vi "Dsc_Board_Man_Dlg.vi"(8 "error in":errorcluster) -> (0 "error out":errorcluster)   [LabVIEW 2014, in "Dsc_Board_Dlg.lvlib"]
uses:
  Dsc_Board_Dlg.lvlib
  <vilib>/Utility/miscctls.llb/LVRowAndColumnTypeDef.ctl
  DataBase/DataBase.lvlib
  DetectElecrodes/DetectElectros.lvlib
panel:
  in  "退出":bool
  in  "删除":bool
  in  "修改":bool
  in  "新增":bool
  in  "采集卡管理":i32(listbox)
  in  "OK":bool
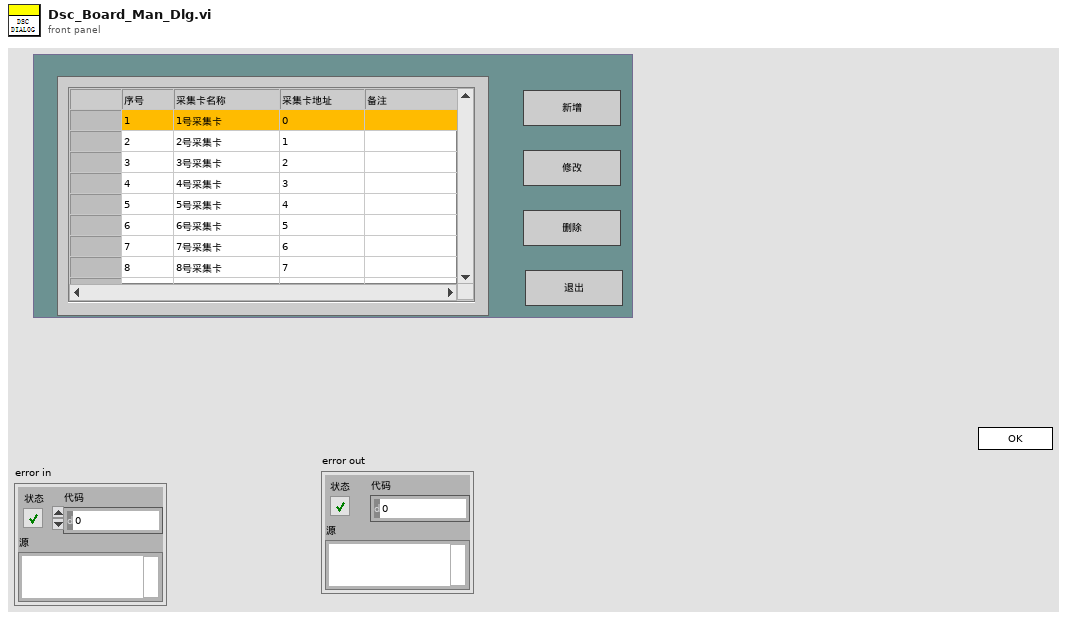
[diagram p1: front panel]
types:
  T1 = enum32{"invalid app kind", "Development System", "Run Time System", "Student Edition", "Embedded LabVIEW", "Evaluation", "Custom"}
  T2 = enum32{"Invalid", "Standard", "Closed", "Hidden", "Minimized", "Maximized"}
  T3 = typedef "LVPoint32TypeDef.ctl" = cluster{"Horizontal":i32, "Vertical":i32}
  T4 = typedef "LVRowAndColumnTypeDef.ctl" = cluster{"Row":i32, "Column":i32}
  T5 = cluster{"Core":cluster{"Current VI Reference":refnum<vi>, "Close Panel on Exit?":bool}, "Your Boolean data":bool, "Your string data":string, "行列":T4}
  T6 = cluster{"Current VI Reference":refnum<vi>, "Close Panel on Exit?":bool}
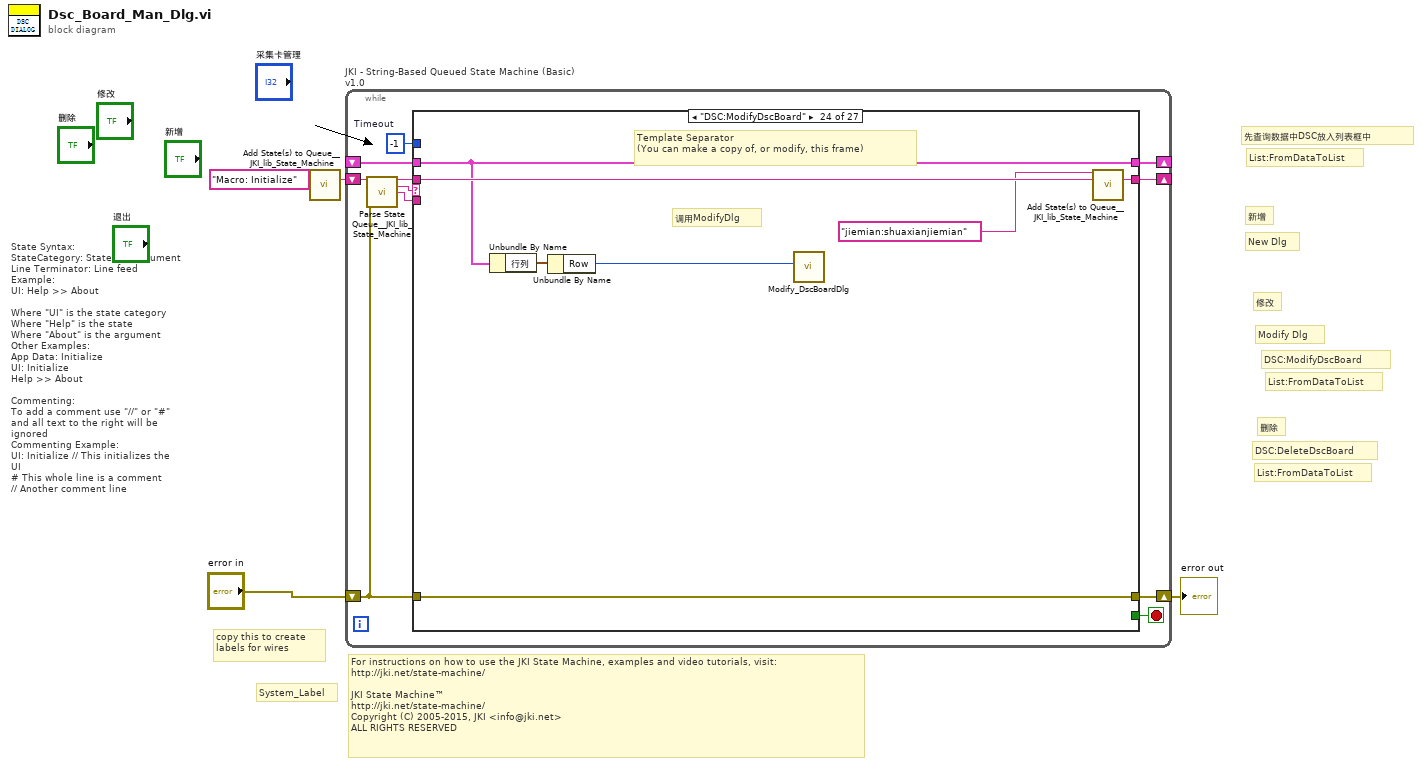
[diagram p0: block diagram]
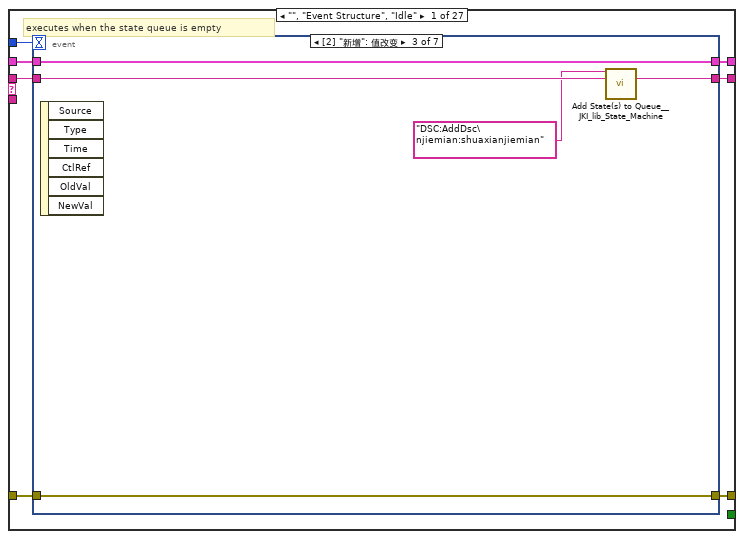
[diagram p2: hidden frame]
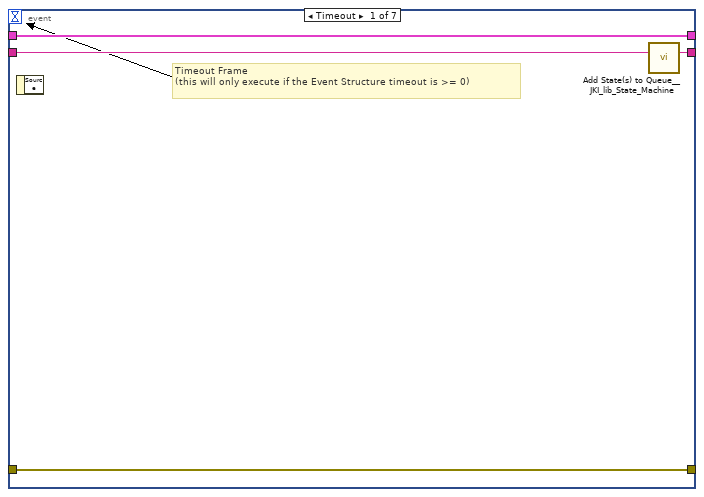
[diagram p3: hidden frame]
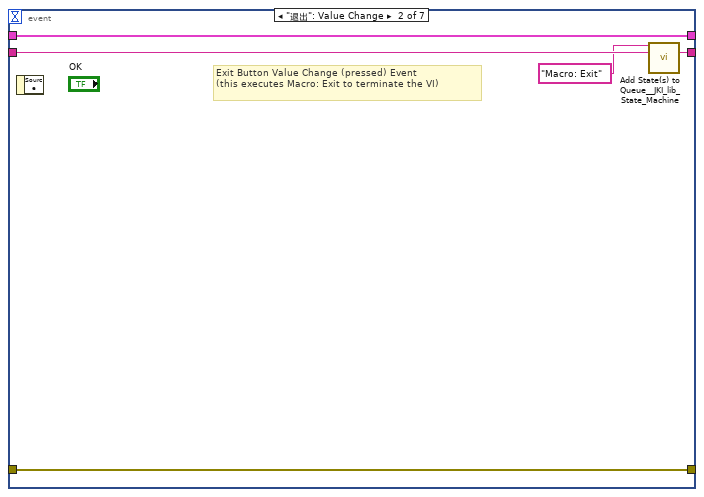
[diagram p4: hidden frame]
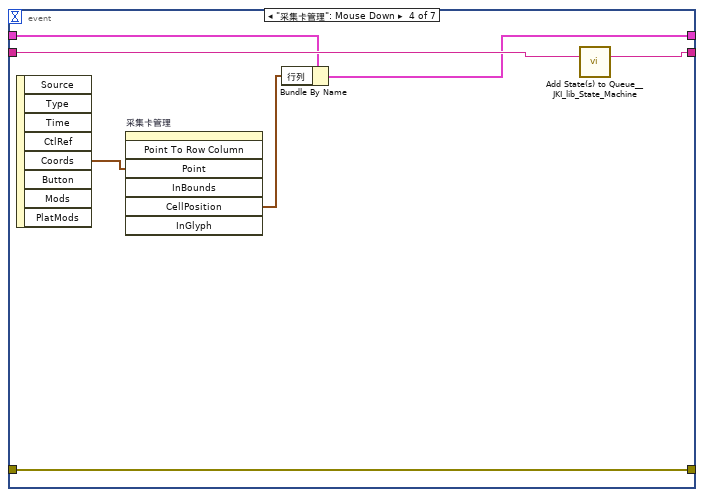
[diagram p5: hidden frame]
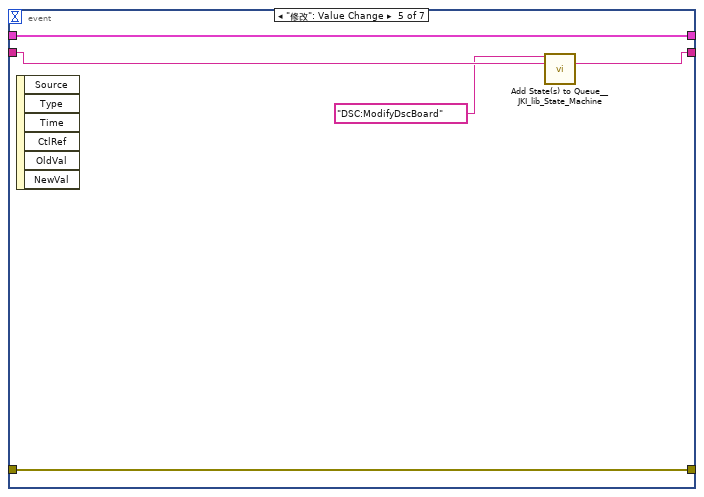
[diagram p6: hidden frame]
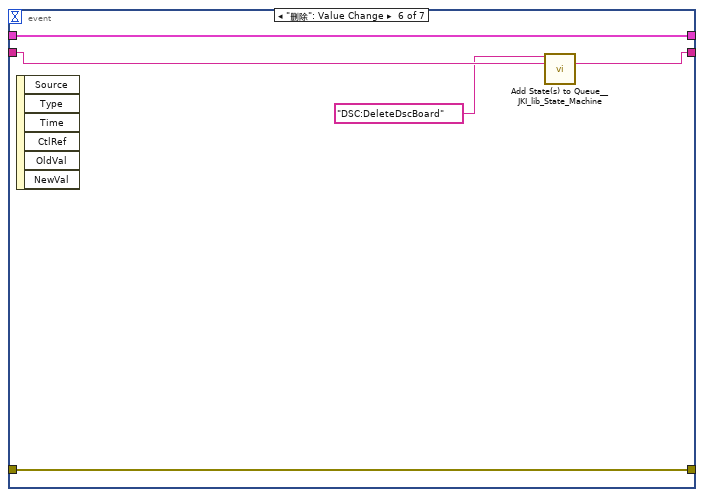
[diagram p7: hidden frame]
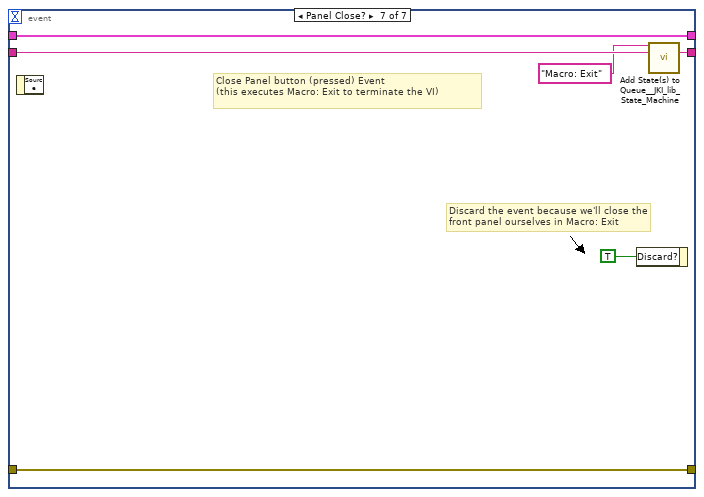
[diagram p8: hidden frame]
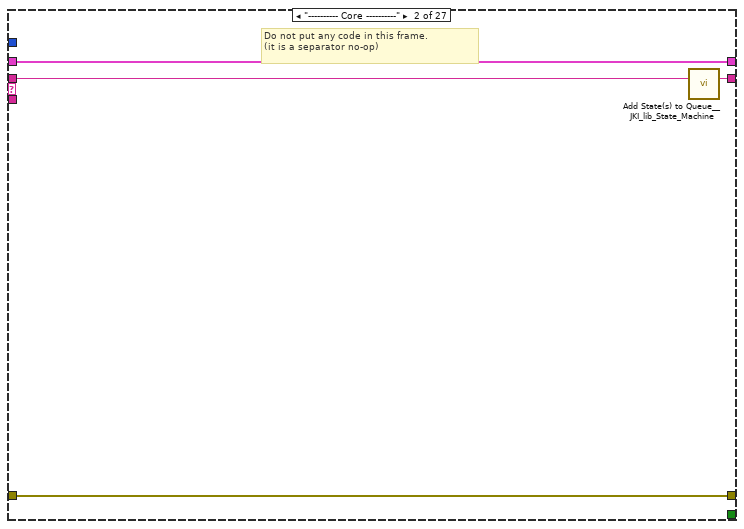
[diagram p9: hidden frame]
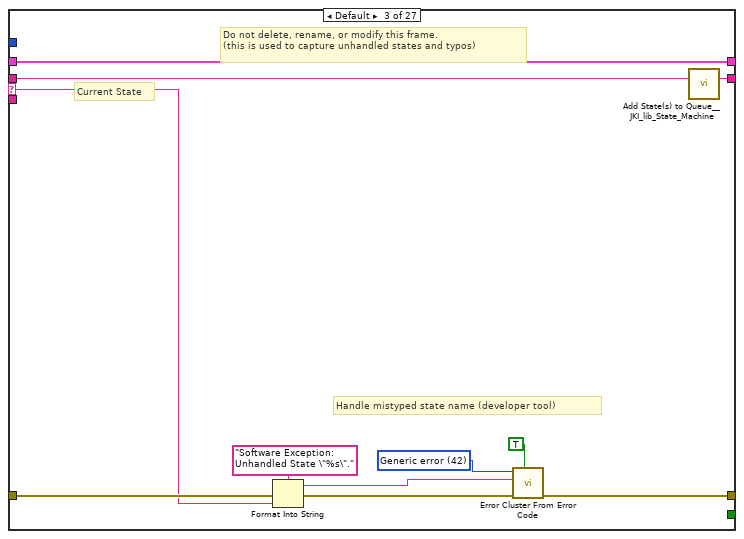
[diagram p10: hidden frame]
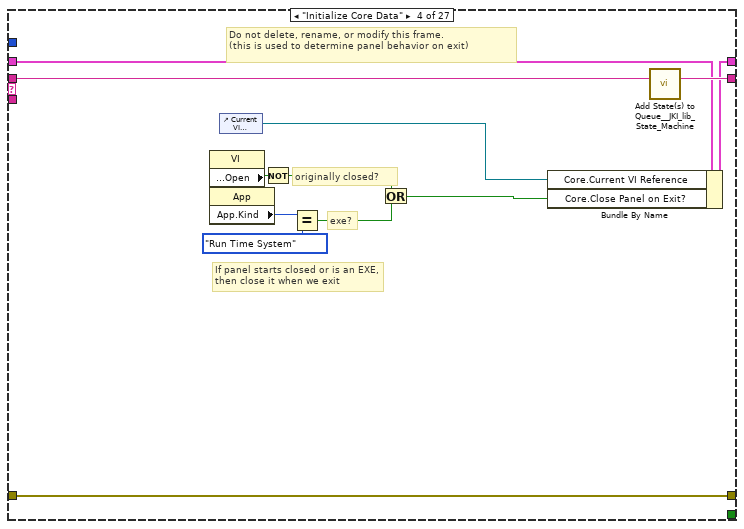
[diagram p11: hidden frame]
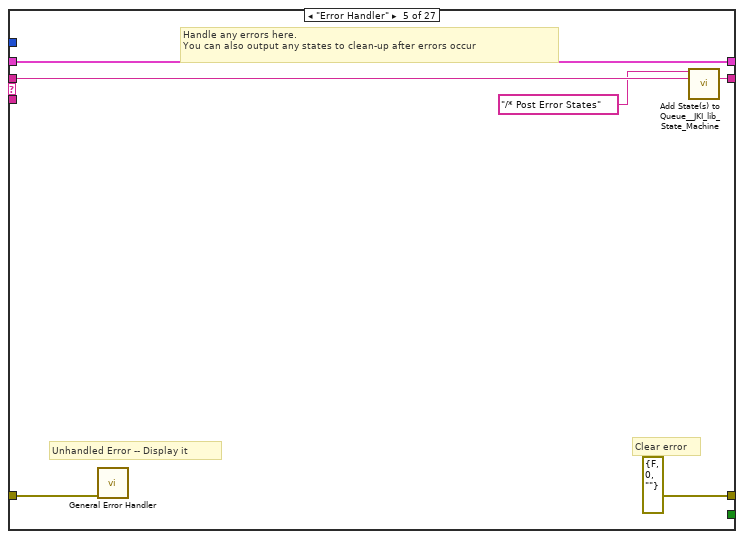
[diagram p12: hidden frame]
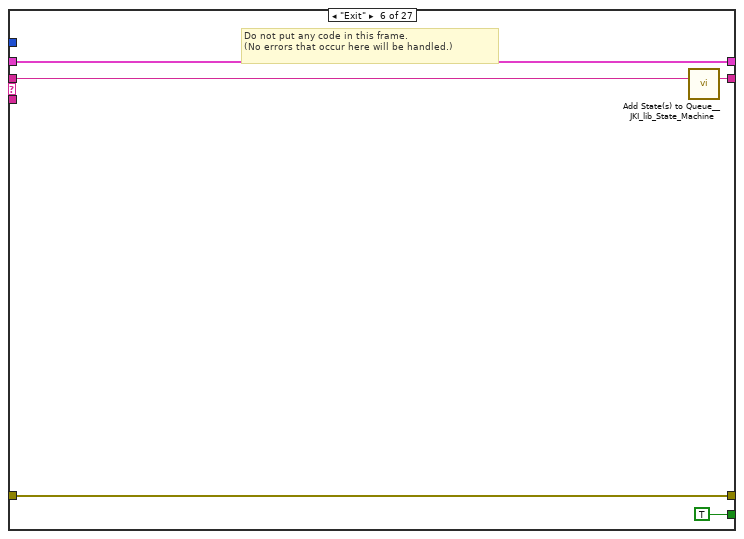
[diagram p13: hidden frame]
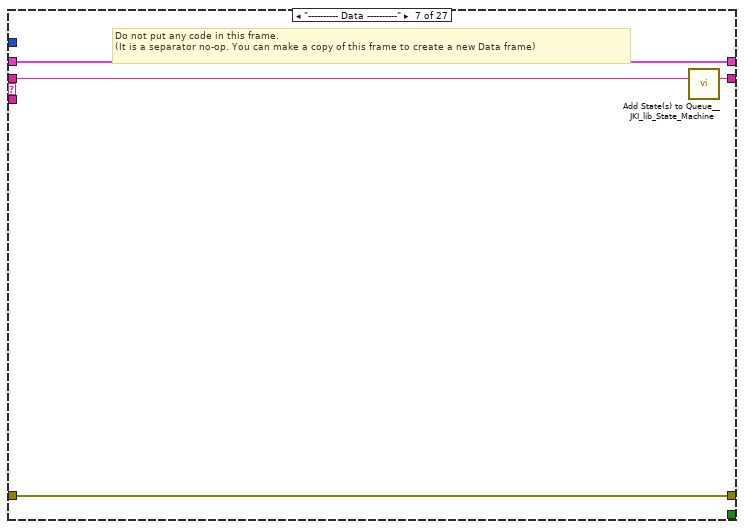
[diagram p14: hidden frame]
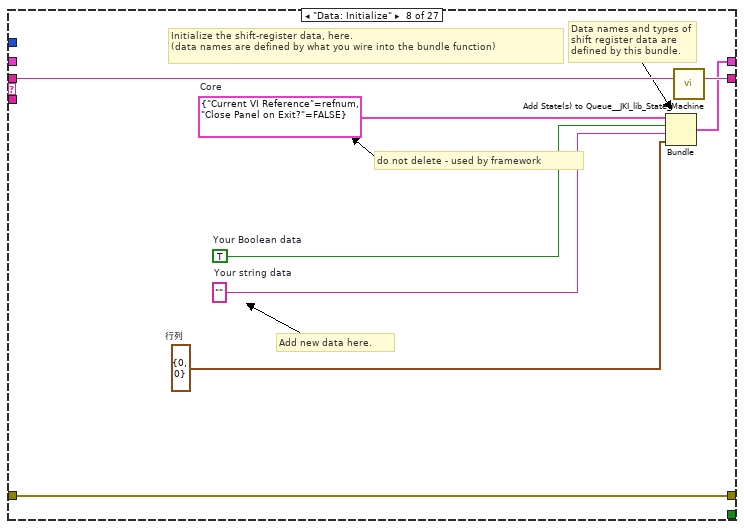
[diagram p15: hidden frame]
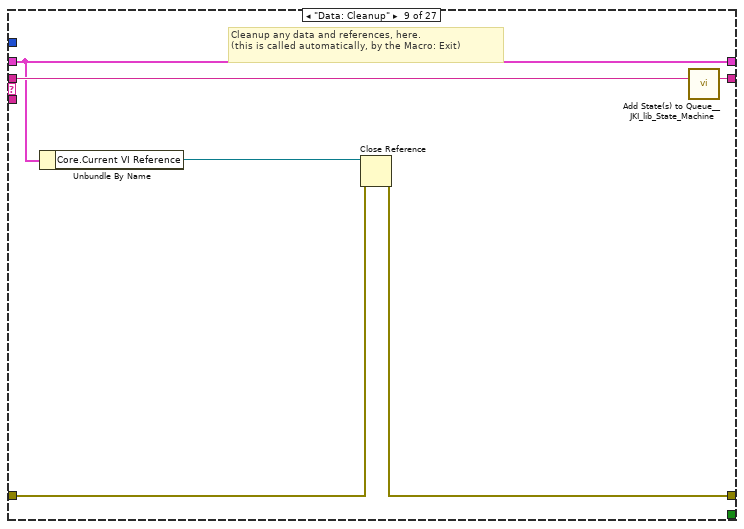
[diagram p16: hidden frame]
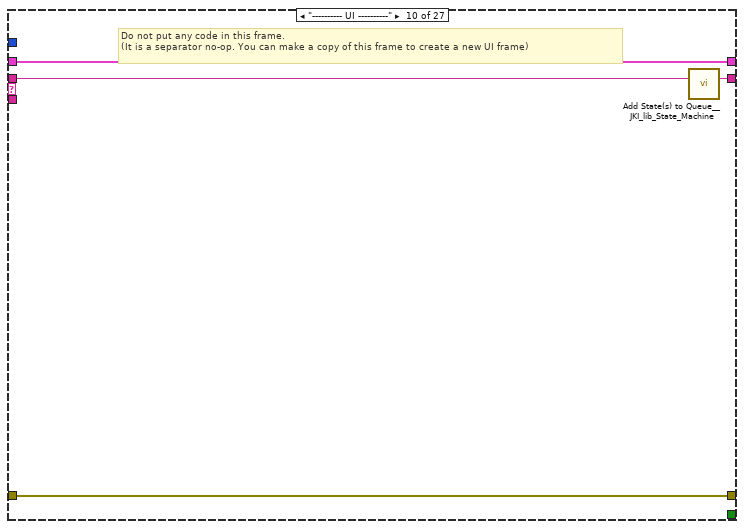
[diagram p17: hidden frame]
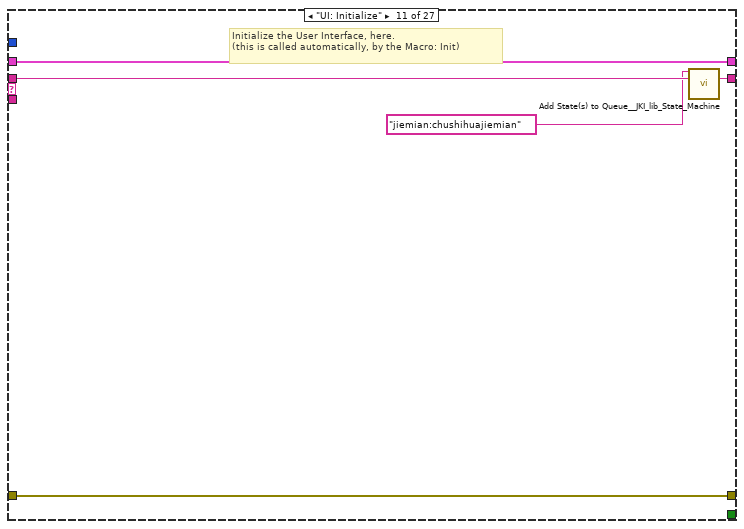
[diagram p18: hidden frame]
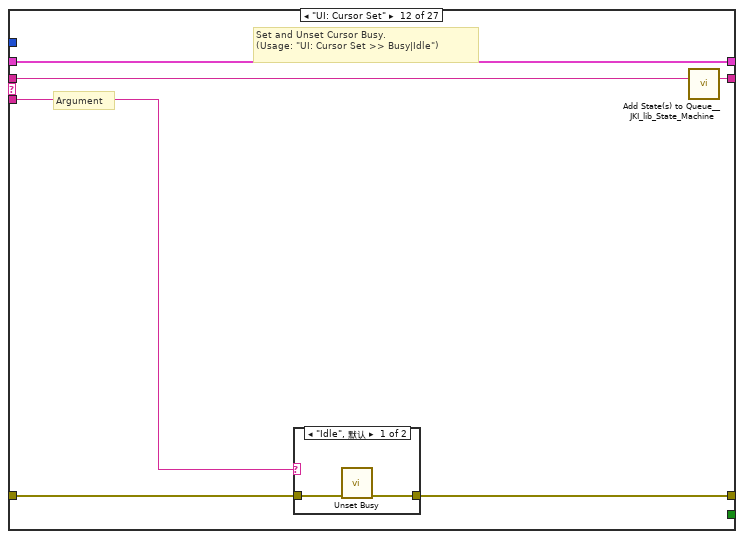
[diagram p19: hidden frame]
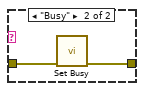
[diagram p20: hidden frame]
diagram:
  # "List:FromDataToList"
  # "DSC:DeleteDscBoard"
  # "删除"
  # "List:FromDataToList"
  # "DSC:ModifyDscBoard"
  # "Modify Dlg"
  # "修改"
  # "New Dlg"
  # "List:FromDataToList"
  # "先查询数据中DSC放入列表框中"
  # "新增"
  # "For instructions on how to use the JKI State Machine, examples and video tutorials, visit:\nhttp://jki.net/state-machine/\n\nJKI State Machine™\nhttp://jki.net/state-machine/\nCopyright (C) 2005-2015, JKI <info@jki.net>\nALL RIGHTS RESERVED"
  # "State Syntax:\nStateCategory: State >> Argument\nLine Terminator: Line feed\nExample:\nUI: Help >> About\n\nWhere \"UI\" is the state category\nWhere \"Help\" is the state\nWhere \"About\" is the argument\nOther Examples:\nApp Data: Initialize\nUI: Initialize\nHelp >> About\n\nCommenting:\nTo add a comment use \"//\" or \"#\" and all text to the right will be ignored\nCommenting Example:\nUI: Initialize // This initializes the UI\n# This whole line is a comment\n// Another comment line"
  # "copy this to create labels for wires"
  # "System_Label"
  n1 = call <vilib>:"Add State(s) to Queue__JKI_lib_State_Machine.vi"("State(s) in (\"\")"="Macro: Initialize") -> ("States Out"=w4:string)  [unwired: 14 in]
  n2 = while "JKI - String-Based Queued State Machine (Basic) v1.0" {
    shift-right: [w8] -> _
    shift-left: _ -> [w7]
    shift-right: [w11] -> w2
    shift-left: "error in" -> [w5]
    shift-right: [w10] -> _
    shift-left: w4 -> [w12]
    stop <- w9 stop-if-true
    w6 = -1  # Timeout
    n3 = call <vilib>:"Parse State Queue__JKI_lib_State_Machine.vi"("State Queue"=w12, "Error In (no error)"=w5) -> ("Remaining States"=w14:string, "Current State"=w15:string, "Arguments"=w13:string)  [unwired: 11 in]
    n4 = case shown="\"DSC:ModifyDscBoard\"" w15 {
      selector: w15 -> [_ _ w64 _ _ _ _ _ _ _ _ _ _ _ _ _ _ _ _ _ _ _ _ _ _ _ _]
      tunnel: w14 -> [w22 w63 w68 w86 w92 w97 w101 w109 w115 w119 w124 w130 w141 w167 w172 w182 w186 w197 w206 w215 w219 w223 w233 w240 w244 w248 w252]
      tunnel: w13 -> [_ _ _ _ _ _ _ _ _ _ _ w125 w135 _ _ _ _ _ _ _ _ _ _ _ _ _ _]
      tunnel: w7 -> [w20 w60 w66 w77 w89 w95 w98 _ w110 w116 w122 w128 w137 w164 w169 w179 w183 w194 w203 w212 w216 w220 w231 w237 w241 w245 w249]
      tunnel: [w19 w61 w70 w83 errorcluster {"status"=FALSE, "code"=0, "source"=""} ("error out") w94 w99 w106 w111 w117 w121 w126 w138 w165 w170 w180 w184 w195 w204 w213 w217 w221 w225 w238 w242 w246 w250] -> w11
      tunnel: w5 -> [w18 w61 w69 w83 w88 w94 w99 w106 w112 w117 w121 w127 w139 w165 w170 w180 w184 w195 w204 w213 w217 w221 w226 w238 w242 w246 w250]
      tunnel: [w21 w62 w67 w85 w91 w96 w100 w108 w114 w118 w123 w129 w140 w166 w171 w181 w185 w196 w205 w214 w218 w222 w232 w239 w243 w247 w251] -> w10
      tunnel: [_ _ _ _ _ TRUE _ _ _ _ _ _ _ _ _ _ _ _ _ _ _ _ _ _ _ _ _] -> w9
      tunnel: [w17 w60 w66 w84 w89 w95 w98 w107 w110 w116 w122 w128 w137 w164 w169 w179 w183 w194 w203 w212 w216 w220 w231 w237 w241 w245 w249] -> w8
      tunnel: w6 -> [w16 _ _ _ _ _ _ _ _ _ _ _ _ _ _ _ _ _ _ _ _ _ _ _ _ _ _]
      frame "", "Event Structure", "Idle" {
        # "executes when the state queue is empty"
        n5 = event shown="[2] \"新增\": 值改变" {
          selector: _ -> [_ _ _ _ _ _ _]
          dyn-events: _ -> [_ _ _ _ _ _ _]
          timeout: w16 -> [_ _ _ _ _ _ _]
          tunnel: w22 -> [w26 w31 w35 w42 w46 w51 w59]
          tunnel: [w25 w30 w36 w43 w48 w53 w58] -> w21
          tunnel: w20 -> [w23 w28 w33 w38 w47 w52 w56]
          tunnel: [w24 w29 w34 w40 w44 w49 w57] -> w19
          tunnel: w18 -> [w24 w29 w34 w40 w44 w49 w57]
          tunnel: [w23 w28 w33 w37 w47 w52 w56] -> w17
          event Timeout {
            # "Timeout Frame\n(this will only execute if the Event Structure timeout is >= 0)"
            n6 = event-data() -> ()  [unwired: 1 in, 1 out]
            n7 = call <vilib>:"Add State(s) to Queue__JKI_lib_State_Machine.vi"("State(s) in (\"\")"=w26) -> ("States Out"=w25:string)  [unwired: 14 in]
          }
          event "退出": Value Change {
            # "Exit Button Value Change (pressed) Event\n(this executes Macro: Exit to terminate the VI)"
            n8 = event-data() -> ()  [unwired: 1 in, 1 out]
            n9 = call <vilib>:"Add State(s) to Queue__JKI_lib_State_Machine.vi"("State(s) in Front (\"\")"="Macro: Exit", "State(s) in (\"\")"=w31) -> ("States Out"=w30:string)  [unwired: 13 in]
          }
          event "新增": Value Change {
            n10 = event-data() -> ()  [unwired: 1 in, 6 out]
            n11 = call <vilib>:"Add State(s) to Queue__JKI_lib_State_Machine.vi"("State(s) in Front (\"\")"="DSC:AddDsc\njiemian:shuaxianjiemian", "State(s) in (\"\")"=w35) -> ("States Out"=w36:string)  [unwired: 13 in]
          }
          event "采集卡管理": Mouse Down {
            n12 = event-data() -> ("Coords"=w41:T3)  [unwired: 1 in, 7 out]
            n13 = invoke on="采集卡管理" class="MCListbox (严格)" method="Point To Row Column"("Point"=w41) -> ("CellPosition"=w39:T4)  [unwired: 6 in, 6 out]
            n14 = Bundle By Name(cluster=w38, "行列"=w39) -> (w37:T5)
            n15 = call <vilib>:"Add State(s) to Queue__JKI_lib_State_Machine.vi"("State(s) in (\"\")"=w42) -> ("States Out"=w43:string)  [unwired: 14 in]
          }
          event "修改": Value Change {
            n16 = event-data() -> ()  [unwired: 1 in, 6 out]
            n17 = call <vilib>:"Add State(s) to Queue__JKI_lib_State_Machine.vi"("State(s) in Front (\"\")"="DSC:ModifyDscBoard", "State(s) in (\"\")"=w46) -> ("States Out"=w48:string)  [unwired: 13 in]
          }
          event "删除": Value Change {
            n18 = event-data() -> ()  [unwired: 1 in, 6 out]
            n19 = call <vilib>:"Add State(s) to Queue__JKI_lib_State_Machine.vi"("State(s) in Front (\"\")"="DSC:DeleteDscBoard", "State(s) in (\"\")"=w51) -> ("States Out"=w53:string)  [unwired: 13 in]
          }
          event Panel Close? {
            # "Discard the event because we'll close the front panel ourselves in Macro: Exit"
            # "Close Panel button (pressed) Event\n(this executes Macro: Exit to terminate the VI)"
            n20 = event-data() -> ()  [unwired: 1 in, 1 out]
            n21 = event-data("Discard?"=TRUE) -> ()  [unwired: 1 in, 1 out]
            n22 = call <vilib>:"Add State(s) to Queue__JKI_lib_State_Machine.vi"("State(s) in Front (\"\")"="Macro: Exit", "State(s) in (\"\")"=w59) -> ("States Out"=w58:string)  [unwired: 13 in]
          }
        }
      }
      frame "---------- Core ----------" {
        # "Do not put any code in this frame.\n(it is a separator no-op)"
        n23 = call <vilib>:"Add State(s) to Queue__JKI_lib_State_Machine.vi"("State(s) in (\"\")"=w63) -> ("States Out"=w62:string)  [unwired: 14 in]
      }
      frame Default {
        w73 = 42 items=["No error", "Argument error", "Memory is full", "Out of zone", "End of file", "File already open", "Generic file I/O error", "File not found", "File permission error", "Disk is full", "Duplicate path", "Too many files open", "System feature not enabled", "Resource file not found", "Cannot add resource", "Resource not found", "Image not found", "Image memory error", "Pen does not exist", "Config type invalid", "Config token not found", "Config parse error", "Config memory error", "Bad external code format", "Bad external code offset", "External code not present", "Null window", "Destroy window error", "Null menu", "Print aborted", "Bad print record", "Print driver error", "Windows error during printing", "Memory error during printing", "Print dialog error", "Generic print error", "Invalid device refnum", "Device not found", "Device parameter error", "Device unit error", "Cannot open device", "Device call aborted", "Generic error", "Cancelled by user", "Object ID too low", "Object ID too high", "Object not in heap", "Unknown heap", "Unknown object (invalid DefProc)", "Unknown object (DefProc not in table)", "Message out of range", "Invalid (null) method", "Unknown message", "Manager call not supported", "Bad address", "Network operation in progress", "Network operation timed out", "Connection is busy", "Network attribute not supported", "Network error", "Address in use", "System out of memory", "Connection aborted", "Connection refused", "Not connected", "Already connected", "Connection closed", "Initialization error (interapplication manager)", "Bad occurrence", "Wait on unbound occurrence handler", "Occurrence queue overflow", "Datalog type conflict", "Unused", "Unrecognized type (interapplication manager)", "Memory corrupt", "Failed to make temporary DLL", "Old CIN version", "Drag socket not found", "Failed to load drop-object", "Failed to register OLE object", "Failed to release OLE object", "Format specifier type mismatch", "Unknown format specifier", "Too few format specifiers", "Too many format specifiers", "Scan failed", "Newer CIN version", "Error converting to variant", "Runtime menu error", "Password tampered", "Variant attribute not found", "Incompatible variant data type", "Event data is not available", "Event Store is not present", "Occurrence is not found", "Event Queue is not created", "Event info is not available", "Refnum passed is NULL", "Error retrieving Class GUID", "Error retrieving CoClass GUID", "Error retrieving TypeLib GUID.", "Bad built application magic bytes.", "Specific driver is different from the specific driver associated with the Logical Name.", "There is no session opened to the class driver.", "Max Error", "MAX - Error with config objects", "MAX - Error loading configuration", "MAX - Group not supported"]
        # "Current State"
        # "Do not delete, rename, or modify this frame.\n(this is used to capture unhandled states and typos)"
        # "Handle mistyped state name (developer tool)"
        n24 = Format Into String(format string="Software Exception: Unhandled State \"%s\"." ("message"), error in=w69, w64) -> (resulting string=w72:string, error out=w71:errorcluster)  [unwired: 1 in]
        n25 = call <vilib>:"Error Cluster From Error Code.vi"("show call chain? (False)"=TRUE, "error in (no error)"=w71, "error message (\"\")"=w72, "error code (0)"=w73) -> ("error out"=w70:errorcluster)  [unwired: 5 in]
        n26 = call <vilib>:"Add State(s) to Queue__JKI_lib_State_Machine.vi"("State(s) in (\"\")"=w68) -> ("States Out"=w67:string)  [unwired: 14 in]
      }
      frame "Initialize Core Data" {
        # "Do not delete, rename, or modify this frame.\n(this is used to determine panel behavior on exit)"
        # "originally closed?"
        # "exe?"
        # "If panel starts closed or is an EXE, then close it when we exit"
        n27 = property class="VI"() -> ("Front Panel.Open"=w82:bool)  [unwired: 2 in, 2 out]
        n28 = property class="App"() -> ("App.Kind"=w81:T1)  [unwired: 2 in, 2 out]
        n29 = control-ref of="Current VI Reference"() -> (w75:refnum<vi>)
        n30 = Not(x=w82) -> (.not. x?=w79:bool)
        n31 = Equal?(x=w81, y=T1."Run Time System" ("Application:Kind")) -> (x = y?=w78:bool)
        n32 = Or(x=w79, y=w78) -> (x .or. y?=w76:bool)
        n33 = Bundle By Name(cluster=w77, "Core.Current VI Reference"=w75, "Core.Close Panel on Exit?"=w76) -> (w84:T5)
        n34 = call <vilib>:"Add State(s) to Queue__JKI_lib_State_Machine.vi"("State(s) in (\"\")"=w86) -> ("States Out"=w85:string)  [unwired: 14 in]
      }
      frame "Error Handler" {
        # "Unhandled Error -- Display it"
        # "Handle any errors here.\nYou can also output any states to clean-up after errors occur"
        # "Clear error"
        n35 = call <vilib>:"General Error Handler.vi"("error in (no error)"=w88) -> ()  [unwired: 10 in, 5 out]
        n36 = call <vilib>:"Add State(s) to Queue__JKI_lib_State_Machine.vi"("State(s) in Front (\"\")"="/* Post Error States", "State(s) in (\"\")"=w92) -> ("States Out"=w91:string)  [unwired: 13 in]
      }
      frame "Exit" {
        # "Do not put any code in this frame.\n(No errors that occur here will be handled.)"
        n37 = call <vilib>:"Add State(s) to Queue__JKI_lib_State_Machine.vi"("State(s) in (\"\")"=w97) -> ("States Out"=w96:string)  [unwired: 14 in]
      }
      frame "---------- Data ----------" {
        # "Do not put any code in this frame.\n(It is a separator no-op. You can make a copy of this frame to create a new Data frame)"
        n38 = call <vilib>:"Add State(s) to Queue__JKI_lib_State_Machine.vi"("State(s) in (\"\")"=w101) -> ("States Out"=w100:string)  [unwired: 14 in]
      }
      frame "Data: Initialize" {
        w102 = T4 {"Row"=0, "Column"=0}  # 行列
        w103 = T6 {"Current VI Reference"=refnum, "Close Panel on Exit?"=FALSE}  # Core
        w105 = TRUE  # Your Boolean data
        w104 = ""  # Your string data
        # "do not delete - used by framework"
        # "Add new data here."
        # "Data names and types of shift register data are defined by this bundle."
        # "Initialize the shift-register data, here.\n(data names are defined by what you wire into the bundle function)"
        n39 = Bundle("Core"=w103, "Your Boolean data"=w105, "Your string data"=w104, "行列"=w102) -> (w107:T5)  [unwired: 1 in]
        n40 = call <vilib>:"Add State(s) to Queue__JKI_lib_State_Machine.vi"("State(s) in (\"\")"=w109) -> ("States Out"=w108:string)  [unwired: 14 in]
      }
      frame "Data: Cleanup" {
        # "Cleanup any data and references, here.\n(this is called automatically, by the Macro: Exit)"
        n41 = Unbundle By Name(w110) -> ("Core.Current VI Reference"=w113:refnum<vi>)
        n42 = Close Reference(reference=w113, error in (no error)=w112) -> (error out=w111:errorcluster)
        n43 = call <vilib>:"Add State(s) to Queue__JKI_lib_State_Machine.vi"("State(s) in (\"\")"=w115) -> ("States Out"=w114:string)  [unwired: 14 in]
      }
      frame "---------- UI ----------" {
        # "Do not put any code in this frame.\n(It is a separator no-op. You can make a copy of this frame to create a new UI frame)"
        n44 = call <vilib>:"Add State(s) to Queue__JKI_lib_State_Machine.vi"("State(s) in (\"\")"=w119) -> ("States Out"=w118:string)  [unwired: 14 in]
      }
      frame "UI: Initialize" {
        # "Initialize the User Interface, here.\n(this is called automatically, by the Macro: Init)"
        n45 = call <vilib>:"Add State(s) to Queue__JKI_lib_State_Machine.vi"("State(s) in Front (\"\")"="jiemian:chushihuajiemian", "State(s) in (\"\")"=w124) -> ("States Out"=w123:string)  [unwired: 13 in]
      }
      frame "UI: Cursor Set" {
        # "Argument"
        # "Set and Unset Cursor Busy.\n(Usage: \"UI: Cursor Set >> Busy|Idle\")"
        n46 = case shown="\"Idle\", 默认" w125 {
          tunnel: w127 -> [w132 w134]
          tunnel: [w131 w133] -> w126
          frame "Idle", Default {
            n47 = call <vilib>:"Unset Busy.vi"("error in (no error)"=w132) -> ("error out"=w131:errorcluster)  [unwired: 10 in]
          }
          frame "Busy" {
            n48 = call <vilib>:"Set Busy.vi"("error in (no error)"=w134) -> ("error out"=w133:errorcluster)  [unwired: 9 in, 1 out]
          }
        }
        n49 = call <vilib>:"Add State(s) to Queue__JKI_lib_State_Machine.vi"("State(s) in (\"\")"=w130) -> ("States Out"=w129:string)  [unwired: 14 in]
      }
      frame "UI: Front Panel State" {
        # "Argument"
        # "Set Front Panel Open or Closed\n(Usage: \"UI: Front Panel State >> Open|Close\")"
        n50 = Unbundle By Name(w137) -> ("Core.Current VI Reference"=w136:refnum<vi>)
        n51 = case shown="\"Open\", 默认" w135 {
          tunnel: w139 -> [w145 w158]
          tunnel: [w147 w159] -> w138
          tunnel: w136 -> [w146 w156]
          frame "Open", Default {
            n52 = property class="VI"(reference=w146, error in=w145) -> (reference out=w143:refnum<vi>, error out=w144:errorcluster, "Front Panel.Open"=w142:bool)
            n53 = case shown="假" w142 {
              tunnel: [w150 w153] -> w147
              tunnel: w144 -> [w149 w153]
              tunnel: w143 -> [w148 _]
              frame False {
                n54 = invoke class="VI" method="FP.Open"(reference=w148, error in=w149, "Activate"=TRUE, "State"=T2."Standard") -> (error out=w150:errorcluster)  [unwired: 1 in, 4 out]
              }
              frame True {
              }
            }
          }
          frame "Close" {
            n55 = property class="VI"(reference=w156, error in=w158) -> (reference out=w155:refnum<vi>, error out=w157:errorcluster, "Front Panel.Open"=w154:bool)
            n56 = case shown="真" w154 {
              tunnel: [w160 w163] -> w159
              tunnel: w157 -> [w160 w162]
              tunnel: w155 -> [_ w161]
              frame False {
              }
              frame True {
                n57 = invoke class="VI" method="FP.Close"(reference=w161, error in=w162) -> (error out=w163:errorcluster)  [unwired: 1 in, 2 out]
              }
            }
          }
        }
        n58 = call <vilib>:"Add State(s) to Queue__JKI_lib_State_Machine.vi"("State(s) in (\"\")"=w141) -> ("States Out"=w140:string)  [unwired: 14 in]
      }
      frame "---------- Macro ----------" {
        # "Do not put any code in this frame.\n(It is a separator no-op. You can make a copy of this frame to create a new Macro frame)"
        n59 = call <vilib>:"Add State(s) to Queue__JKI_lib_State_Machine.vi"("State(s) in (\"\")"=w167) -> ("States Out"=w166:string)  [unwired: 14 in]
      }
      frame "Macro: Initialize" {
        w168 = "Data: Initialize\nInitialize Core Data\nUI: Initialize\nUI: Front Panel State >> Open"  # Data: Initialize Initialize Core Data UI: Initialize UI: Front Panel State >> Open
        # "Initialization Macro\n(This is called once, when the VI starts)"
        n60 = call <vilib>:"Add State(s) to Queue__JKI_lib_State_Machine.vi"("State(s) in Front (\"\")"=w168, "State(s) in (\"\")"=w172) -> ("States Out"=w171:string)  [unwired: 13 in]
      }
      frame "Macro: Exit" {
        # "Exit Macro\n(This is called once, when the VI exits)"
        n61 = Unbundle By Name(w179) -> ("Core.Close Panel on Exit?"=w178:bool)
        n62 = Select(t="UI: Front Panel State >> Close", s=w178, f="") -> (s? t:f=w175:string)
        n63 = call <vilib>:"Add State(s) to Queue__JKI_lib_State_Machine.vi"("State(s) in (\"\")"=w175, "State(s) at Back (\"\")"="Data: Cleanup\nExit") -> ("States Out"=w173:string)  [unwired: 13 in]
        n64 = call <vilib>:"Add State(s) to Queue__JKI_lib_State_Machine.vi"("State(s) in Front (\"\")"=w173, "State(s) in (\"\")"=w182) -> ("States Out"=w181:string)  [unwired: 13 in]
      }
      frame "------------------List---------------" {
        # "Template Separator\n(You can make a copy of, or modify, this frame)"
        n65 = call <vilib>:"Add State(s) to Queue__JKI_lib_State_Machine.vi"("State(s) in (\"\")"=w186) -> ("States Out"=w185:string)  [unwired: 14 in]
      }
      frame "List:FromDataToList" {
        (unwired) "select *from t_dsc_board order by dsc_board_address asc;"
        # "先查询数据中DSC放入列表框中"
        # "Template Separator\n(You can make a copy of, or modify, this frame)"
        n66 = call "SelectData.vi"("SQL query"="select *from t_dsc_board;") -> ("recordset data"=w192:variant[][])  [unwired: 7 in, 1 out]
        n67 = call "ReadDataFromDatabase.vi"("长度"=4, "index"=0, "recordset data"=w192) -> ("所有记录"=w189:string[][])  [unwired: 7 in, 1 out]
        n68 = Array Subset(array=w189, index (col)=1 ("索引")) -> (w187:string[][])  [unwired: 3 in]
        n69 = property on="采集卡管理" class="MCListbox (严格)"("ItemNames"=w187) -> ()  [unwired: 2 in, 2 out]
        n70 = call <vilib>:"Add State(s) to Queue__JKI_lib_State_Machine.vi"("State(s) in (\"\")"=w197) -> ("States Out"=w196:string)  [unwired: 14 in]
      }
      frame "jiemian:chushihuajiemian" {
        (unwired) "select *from t_dsc_board order by dsc_board_address asc;"
        (unwired) 1 ("索引")
        # "先查询数据中DSC放入列表框中"
        # "Template Separator\n(You can make a copy of, or modify, this frame)"
        n71 = call "SelectData.vi"("SQL query"="select *from t_dsc_board;") -> ("recordset data"=w201:variant[][])  [unwired: 7 in, 1 out]
        n72 = call "ReadDataFromDatabase.vi"("长度"=4, "index"=0, "recordset data"=w201) -> ("所有记录"=w198:string[][])  [unwired: 7 in, 1 out]
        n73 = property on="采集卡管理" class="MCListbox (严格)"("ItemNames"=w198) -> ()  [unwired: 2 in, 2 out]
        n74 = call <vilib>:"Add State(s) to Queue__JKI_lib_State_Machine.vi"("State(s) in (\"\")"=w206) -> ("States Out"=w205:string)  [unwired: 14 in]
      }
      frame "jiemian:shuaxianjiemian" {
        (unwired) "select *from t_dsc_board order by dsc_board_address asc;"
        # "先查询数据中DSC放入列表框中"
        # "Template Separator\n(You can make a copy of, or modify, this frame)"
        n75 = call "SelectData.vi"("SQL query"="select *from t_dsc_board;") -> ("recordset data"=w210:variant[][])  [unwired: 7 in, 1 out]
        n76 = call "ReadDataFromDatabase.vi"("长度"=4, "index"=0, "recordset data"=w210) -> ("所有记录"=w207:string[][])  [unwired: 7 in, 1 out]
        n77 = property on="采集卡管理" class="MCListbox (严格)"("ItemNames"=w207) -> ()  [unwired: 2 in, 2 out]
        n78 = call <vilib>:"Add State(s) to Queue__JKI_lib_State_Machine.vi"("State(s) in (\"\")"=w215) -> ("States Out"=w214:string)  [unwired: 14 in]
      }
      frame "----------DSC---------" {
        # "Template Separator\n(You can make a copy of, or modify, this frame)"
        n79 = call <vilib>:"Add State(s) to Queue__JKI_lib_State_Machine.vi"("State(s) in (\"\")"=w219) -> ("States Out"=w218:string)  [unwired: 14 in]
      }
      frame "DSC:AddDsc" {
        # "Template Separator\n(You can make a copy of, or modify, this frame)"
        n80 = call "New_DscBoardDlg.vi"() -> ()  [unwired: 12 in]
        n81 = call <vilib>:"Add State(s) to Queue__JKI_lib_State_Machine.vi"("State(s) in (\"\")"=w223) -> ("States Out"=w222:string)  [unwired: 14 in]
      }
      frame "DSC:DeleteDscBoard" {
        # "Template Separator\n(You can make a copy of, or modify, this frame)"
        n82 = Unbundle By Name(w231) -> ("行列.Row"=w228:i32)
        n83 = Number To Decimal String(number=w228) -> (decimal integer string=w229:string)  [unwired: 1 in]
        n84 = Format Into String(format string="delete from t_dsc_board \nwhere dsc_board_id\n=(select tbd.dsc_board_id from \n(select dsc_board_id from t_dsc_board limit %s,1) tbd);", w229) -> (resulting string=w227:string)  [unwired: 2 in, 1 out]
        n85 = call "deleteData.vi"("error in"=w226, "SQL query"=w227) -> ("error out"=w225:errorcluster)  [unwired: 9 in]
        n86 = call <vilib>:"Add State(s) to Queue__JKI_lib_State_Machine.vi"("State(s) in Front (\"\")"="jiemian:shuaxianjiemian", "State(s) in (\"\")"=w233) -> ("States Out"=w232:string)  [unwired: 13 in]
      }
      frame "DSC:ModifyDscBoard" {
        # "调用ModifyDlg"
        # "Template Separator\n(You can make a copy of, or modify, this frame)"
        n87 = Unbundle By Name(w237) -> ("行列"=w236:T4)
        n88 = Unbundle By Name(w236) -> ("Row"=w235:i32)
        n89 = call "Modify_DscBoardDlg.vi"("序号"=w235) -> ()  [unwired: 11 in]
        n90 = call <vilib>:"Add State(s) to Queue__JKI_lib_State_Machine.vi"("State(s) in Front (\"\")"="jiemian:shuaxianjiemian", "State(s) in (\"\")"=w240) -> ("States Out"=w239:string)  [unwired: 13 in]
      }
      frame "---------- New Category ----------" {
        # "Template Separator\n(You can make a copy of, or modify, this frame)"
        n91 = call <vilib>:"Add State(s) to Queue__JKI_lib_State_Machine.vi"("State(s) in (\"\")"=w244) -> ("States Out"=w243:string)  [unwired: 14 in]
      }
      frame "New Category: 1" {
        # "Your code here.\n(You can make a copy of, or modify, this frame)"
        n92 = call <vilib>:"Add State(s) to Queue__JKI_lib_State_Machine.vi"("State(s) in (\"\")"=w248) -> ("States Out"=w247:string)  [unwired: 14 in]
      }
      frame "New Category: 2" {
        # "Your code here.\n(You can make a copy of, or modify, this frame)"
        n93 = call <vilib>:"Add State(s) to Queue__JKI_lib_State_Machine.vi"("State(s) in (\"\")"=w252) -> ("States Out"=w251:string)  [unwired: 14 in]
      }
    }
  }
  "error out" <- w2
